vi "uTTA_ucf_ReadFile_Array.vi"(8 "error in":errorcluster, 11 "selected path":path) -> (0 "error out":errorcluster, 1 "uTTA_CalData":T1(array[cluster]), 2 "TC_Channels":T2(array[cluster]), 3 "TSP_Channels":T2(array[cluster]))   [LabVIEW 2021]
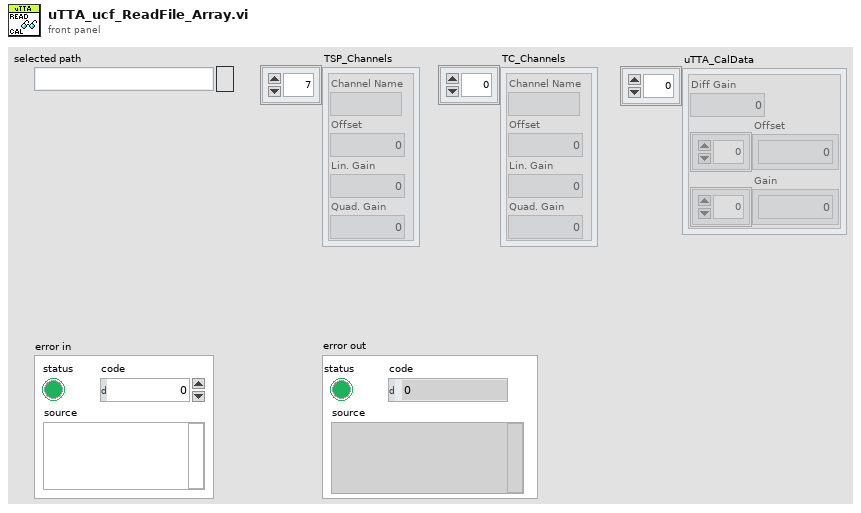
[diagram p1: front panel]
types:
  T1 = cluster{"Diff Gain":dbl, "Offset":dbl[], "Gain":dbl[]}[]
  T2 = cluster{"Channel Name":string, "Offset":dbl, "Lin. Gain":dbl, "Quad. Gain":dbl}[]
  T3 = cluster{"Diff Gain":dbl, "Offset":dbl[], "Gain":dbl[]}
  T4 = typedef "CTL_uTTA_BlockDiagCal.ctl" = cluster{"CH0 Diff Gain":dbl, "Voffs0 Gain":dbl, "CH1 Diff Gain":dbl, "CH2 Diff Gain":dbl, "CH3 Diff Gain":dbl, "Voffs0 Offset":dbl, "Voffs1 Gain":dbl, "Voffs1 Offset":dbl, "CH1 PA0 Gain":dbl, "CH1 PA0 Offset":dbl, "CH2 PA0 Gain":dbl, "CH2 PA0 Offset":dbl, "CH3 PA0 Gain":dbl, "CH3 PA0 Offset":dbl, "CH0 PA0 Gain":dbl, "CH0 PA0 Offset":dbl, "CH0 PA1 Gain":dbl, "CH0 PA1 Offset":dbl, "CH0 PA2 Gain":dbl, "CH0 PA2 Offset":dbl, "CH0 PA3 Gain":dbl, "CH0 PA3 Offset":dbl, "CH_I Gain":dbl, "CH_I Offset":dbl, "I_Sense Gain":dbl, "I_Sense Offset":dbl}
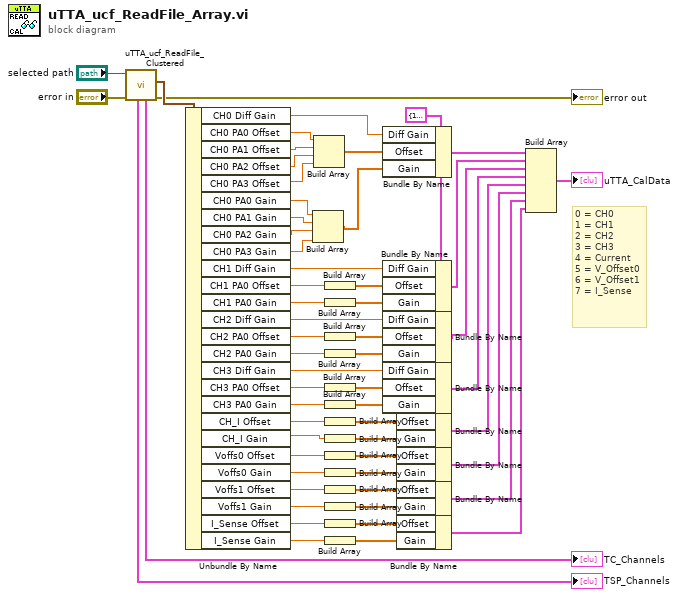
[diagram p0: block diagram]
diagram:
  w19 = T3 {"Diff Gain"=1.0, "Offset"=[], "Gain"=[]}
  # "0 = CH0\n1 = CH1\n2 = CH2\n3 = CH3\n4 = Current\n5 = V_Offset0\n6 = V_Offset1\n7 = I_Sense"
  n1 = call "uTTA_ucf_ReadFile_Clustered.vi"("error in (no error)"="error in", "selected path"="selected path") -> ("error out"=→"error out":errorcluster, "uTTA_Cal"=w4:T4, "TC_Channels"=→"TC_Channels":T2, "TSP_Channels"=→"TSP_Channels":T2)  [unwired: 5 in, 1 out]
  n2 = Unbundle By Name(w4) -> ("CH0 Diff Gain"=w58:dbl, "CH0 PA0 Offset"=w57:dbl, "CH0 PA1 Offset"=w56:dbl, "CH0 PA2 Offset"=w55:dbl, "CH0 PA3 Offset"=w54:dbl, "CH0 PA0 Gain"=w53:dbl, "CH0 PA1 Gain"=w52:dbl, "CH0 PA2 Gain"=w51:dbl, "CH0 PA3 Gain"=w50:dbl, "CH1 Diff Gain"=w46:dbl, "CH1 PA0 Offset"=w45:dbl, "CH1 PA0 Gain"=w43:dbl, "CH2 Diff Gain"=w40:dbl, "CH2 PA0 Offset"=w39:dbl, "CH2 PA0 Gain"=w38:dbl, "CH3 Diff Gain"=w35:dbl, "CH3 PA0 Offset"=w34:dbl, "CH3 PA0 Gain"=w33:dbl, "CH_I Offset"=w22:dbl, "CH_I Gain"=w21:dbl, "Voffs0 Offset"=w25:dbl, "Voffs0 Gain"=w30:dbl, "Voffs1 Offset"=w27:dbl, "Voffs1 Gain"=w26:dbl, "I_Sense Offset"=w17:dbl, "I_Sense Gain"=w16:dbl)
  n3 = Build Array(w53, w52, w51, w50) -> (w48:dbl[])
  n4 = Build Array(w57, w56, w55, w54) -> (w49:dbl[])
  n5 = Build Array(w45) -> (w47:dbl[])
  n6 = Build Array(w43) -> (w44:dbl[])
  n7 = Build Array(w39) -> (w41:dbl[])
  n8 = Build Array(w38) -> (w42:dbl[])
  n9 = Build Array(w34) -> (w37:dbl[])
  n10 = Build Array(w33) -> (w36:dbl[])
  n11 = Build Array(w22) -> (w24:dbl[])
  n12 = Build Array(w21) -> (w23:dbl[])
  n13 = Build Array(w25) -> (w31:dbl[])
  n14 = Build Array(w30) -> (w32:dbl[])
  n15 = Build Array(w27) -> (w29:dbl[])
  n16 = Build Array(w26) -> (w28:dbl[])
  n17 = Build Array(w17) -> (w18:dbl[])
  n18 = Build Array(w16) -> (w20:dbl[])
  n19 = Bundle By Name(cluster=w19, "Diff Gain"=w58, "Offset"=w49, "Gain"=w48) -> (w15:T3)
  n20 = Bundle By Name(cluster=w19, "Diff Gain"=w46, "Offset"=w47, "Gain"=w44) -> (w14:T3)
  n21 = Bundle By Name(cluster=w19, "Diff Gain"=w40, "Offset"=w41, "Gain"=w42) -> (w13:T3)
  n22 = Bundle By Name(cluster=w19, "Diff Gain"=w35, "Offset"=w37, "Gain"=w36) -> (w12:T3)
  n23 = Bundle By Name(cluster=w19, "Offset"=w24, "Gain"=w23) -> (w11:T3)
  n24 = Bundle By Name(cluster=w19, "Offset"=w31, "Gain"=w32) -> (w10:T3)
  n25 = Bundle By Name(cluster=w19, "Offset"=w29, "Gain"=w28) -> (w9:T3)
  n26 = Bundle By Name(cluster=w19, "Offset"=w18, "Gain"=w20) -> (w8:T3)
  n27 = Build Array(w15, w14, w13, w12, w11, w10, w9, w8) -> (→"uTTA_CalData":T1)
